vi "Variant Array Size.vi"(8 "error in (no error)":errorcluster, 11 "data":variant) -> (0 "error out":errorcluster, 2 "is_array?":bool=TRUE, 3 "lengths":i32[](array[numeric]))   [LabVIEW 2021, in "DataTypes_CIF_U.lvlib"]
doc: "Retrieve the dimensions of a variant containing an array."
uses:
  DataTypes_CIF_U.lvlib
  <vilib>/Utility/Data Type/NI_Data Type.lvlib
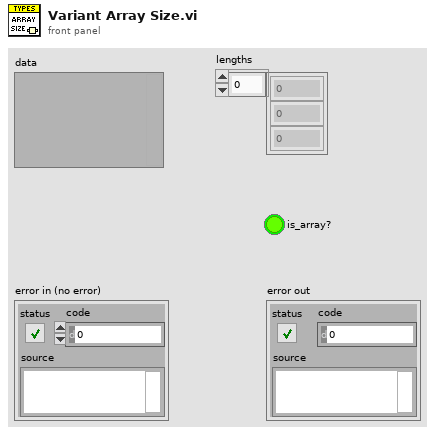
[diagram p1: front panel]
types:
  T1 = typedef "NI_Data Type.lvlib/Data Type.ctl" = enum8{"Invalid Type", "Void", "I8", "I16", "I32", "I64", "U8", "U16", "U32", "U64", "Single Float", "Double Float", "Extended Float", "Single Complex", "Double Complex", "Extended Complex", "Enum U8", "Enum U16", "Enum U32", "Enum U64", "Single Float With Unit", "Double Float With Unit", "Extended Float With Unit", "Single Complex with Unit", "Double Complex with Unit", "Extended Complex with Unit", "Boolean", "String", "Path", "Picture", "Tag", "Array", "Cluster", "Variant", "LV Variant", "Waveform", "Timestamp", "Digital Waveform", "Digital Data", "ExpressData", "Refnum", "External Data", "VI", "Poly VI", "LabVIEW Class Instance", "Fixed Point", "Set Collection", "Map Collection"}
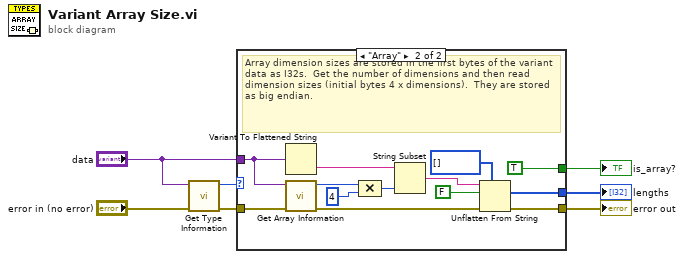
[diagram p0: block diagram]
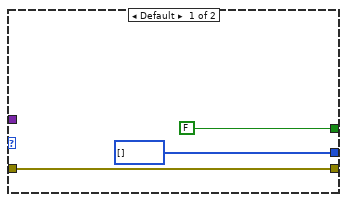
[diagram p2: hidden frame]
diagram:
  n1 = call <vilib>:"Get Type Information.vi"("error in (no error)"="error in (no error)", "variant"="data") -> ("error out"=w4:errorcluster, "type"=w3:T1)  [unwired: 5 in, 3 out]
  n2 = case shown="\"Array\"" w3 {
    tunnel: [i32[] [] w12] -> w7
    tunnel: [w9 w11] -> w6
    tunnel: w4 -> [w9 w23]
    tunnel: [FALSE ("is_array?") TRUE ("is_array?")] -> w2
    tunnel: "data" -> [_ w21]
    frame Default {
    }
    frame "Array" {
      # "Array dimension sizes are stored in the first bytes of the variant data as I32s.  Get the number of dimensions and then read dimension sizes (initial bytes 4 x dimensions).  They are stored as big endian."
      n3 = Variant To Flattened String(Variant=w21) -> (data string=w19:string)  [unwired: 1 out]
      n4 = call <vilib>:"Get Array Information.vi"("error in (no error)"=w23, "variant"=w21) -> ("error out"=w13:errorcluster, "number of dimensions"=w17:i32)  [unwired: 6 in, 2 out]
      n5 = Compound Arithmetic op=MULTIPLY(w17, 4 ("value")) -> (w16:i32)
      n6 = String Subset(string=w19, length (rest)=w16) -> (substring=w18:string)  [unwired: 1 in]
      n7 = Unflatten From String(type=i32[] [] ("initialized array"), binary string=w18, data includes array or string size? (T)=FALSE, error in (no error)=w13) -> (value=w12:i32[], error out=w11:errorcluster)  [unwired: 1 in, 1 out]
    }
  }
  "error out" <- w6
  "lengths" <- w7
  "is_array?" <- w2
